vi "RSNRPZ Configure Corrections.vi"(0 "VISA session":refnum<visa-resource-name> caption="VISA resource name", 1 "Reserved 1 (False)":bool, 2 "Reserved 2 (\"Table 1\")":string="Table 1", 5 "Channel (1)":i32=1, 7 "Offset State (F: Off)":bool, 9 "Offset (0.0 dB)":dbl format="%.2p", 11 "error in (no error)":errorcluster, 12 "S-Parameter Enable (F: Off)":bool) -> (4 "dup VISA session":refnum<visa-resource-name> caption="VISA resource name", 15 "error out":errorcluster)   [LabVIEW 2010]
doc: "This VI configures all correction parameters.\n\nRemote-control command(s):\nSENS:CORR:OFFS\nSENS:CORR:OFFS:STAT ON | OFF\nSENS:CORR:SPD:STAT ON | OFF"
uses:
  rsnrpz_32.dll
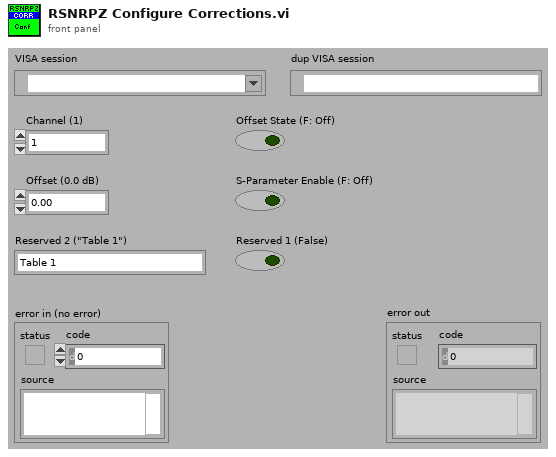
[diagram p1: front panel]
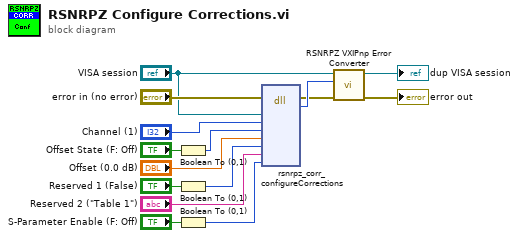
[diagram p0: block diagram]
diagram:
  n1 = Boolean To (0,1)(Boolean="Offset State (F: Off)") -> (0, 1=w10:i16)
  n2 = Boolean To (0,1)(Boolean="Reserved 1 (False)") -> (0, 1=w8:i16)
  n3 = Boolean To (0,1)(Boolean="S-Parameter Enable (F: Off)") -> (0, 1=w6:i16)
  n4 = dll-call lib="rsnrpz_32.dll" fn="rsnrpz_corr_configureCorrections"(error in="error in (no error)", "VISA Session"="VISA session", "Channel"="Channel (1)", "Offset State"=w10, "Offset"="Offset (0.0 dB)", "Offset Table State"=w8, "Table Name"="Reserved 2 (\"Table 1\")", "S-Parameter Enable"=w6) -> (error out=w5:errorcluster, "Status"=w12:i32)  [unwired: 9 in, 1 out]
  n5 = call <instrlib>:"RSNRPZ VXIPnp Error Converter.vi"("error in"=w5, "VXIPnp error code"=w12, "VISA session"="VISA session") -> ("error out"=→"error out":errorcluster, "dup VISA session"=→"dup VISA session":refnum<visa-resource-name>)  [unwired: 7 in]
